vi "Reset Test Time.vi"(10 "Run Queue":set{string}(c389), 11 "Result Model in":refnum<class "Result Model.lvclass">) -> ()   [LabVIEW 2020, in "Result Model.lvclass"]
uses:
  Result Model.lvclass
  Result Model.lvclass/Result Model.ctl
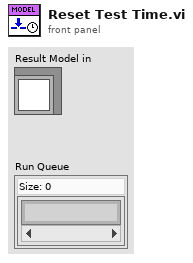
[diagram p1: front panel]
types:
  T1 = typedef "Result Model.lvclass/Model State.ctl" = cluster{"Run Queue":set{string}, "Test Statuses":map{string, T2}, "Execution Time":map{string, dbl}, "Assertions":map{string, cluster{"Result Type":T3, "Status":T2, "Message":string, "Description":string}[]}}
  T2 = typedef "Result.lvlib/Status.ctl" = enum16{"", "Passed", "Failed", "Error", "Skipped", "Setup Error", "Broken", "Teardown Error"}
  T3 = typedef "Result.lvlib/Type.ctl" = enum16{"Method", "Case", "Suite", "Pass", "Fail", "Skip", "Pass if", "Fail if", "Pass if Error", "Fail if Error", "Pass if Equal", "Fail if Equal"}
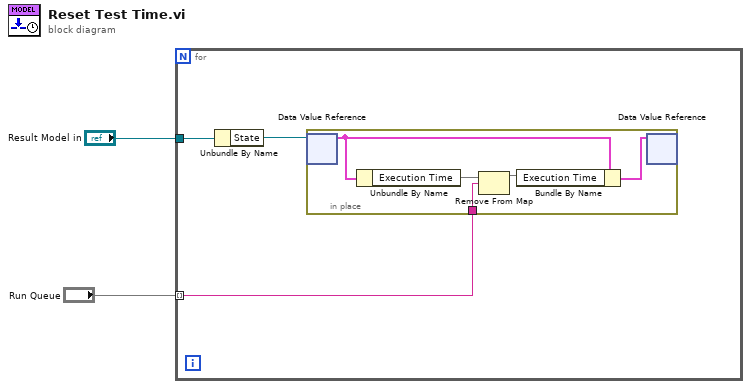
[diagram p0: block diagram]
diagram:
  n1 = for {
    tunnel: "Result Model in" -> [w5]
    tunnel: "Run Queue" -> [w4] mode=indexing
    n2 = Unbundle By Name(w5) -> ("State"=w3:refnum<data-value>)
    n3 = in-place {
      in-place-border: w4 -> [w6]
      n4 = in-place-dvr #1(w3) -> (w9:T1)  [unwired: 1 out]
      n5 = Unbundle By Name(w9) -> ("Execution Time"=w8:map{string, dbl})
      n6 = Remove From Map(10:w6, 11:w8) -> (3:w7:map{string, dbl})  [unwired: 2 out]
      n7 = Bundle By Name(cluster=w9, "Execution Time"=w7) -> (w10:T1)
      n8 = in-place-dvr #1(w10) -> ()  [unwired: 2 out]
    }
  }
